vi "PulseOutput.vi"(1 "Pulse Duration (ms)":u32, 2 "Instantaneous Trigger":bool) -> (0 "State Out":bool)   [LabVIEW 2018]
doc: "This VI produces a True pulse of a specified duration when triggered. The external trigger is expected to be instaneous (e.g. from a rising edge trigger). If the trigger is not instantaneous, the pulse will go True immediately but the pulse timmer will not start counting down until the falling edge of the trigger."
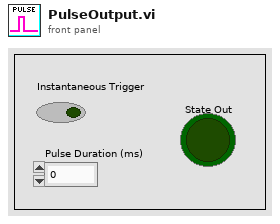
[diagram p1: front panel]
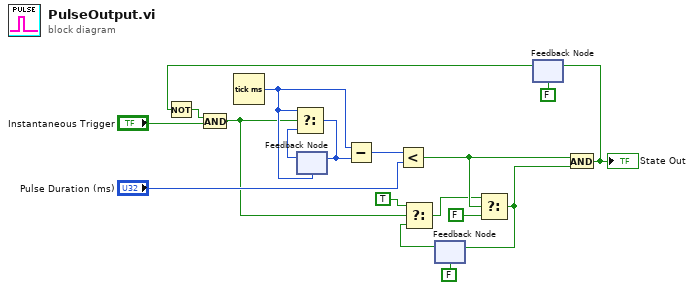
[diagram p0: block diagram]
diagram:
  n1 = Tick Count (ms)() -> (millisecond timer value=w8:u32)
  n2 = feedback #1(w8) -> (w18:u32)
  n3 = feedback #2(FALSE ("f")) -> (w11:bool)
  n4 = feedback #3(FALSE) -> (w2:bool)
  n5 = Not(x=w2) -> (.not. x?=w3:bool)
  n6 = And(x=w3, y="Instantaneous Trigger") -> (x .and. y?=w5:bool)
  n7 = Select(t=w8, s=w5, f=w18) -> (s? t:f=w7:u32)
  n8 = feedback-in #1(w7) -> ()
  n9 = Subtract(x=w8, y=w7) -> (x-y=w17:u32)
  n10 = Less?(x=w17, y="Pulse Duration (ms)") -> (x < y?=w14:bool)
  n11 = Select(t=TRUE, s=w5, f=w11) -> (s? t:f=w13:bool)
  n12 = Select(t=w13, s=w14, f=FALSE) -> (s? t:f=w9:bool)
  n13 = feedback-in #2(w9) -> ()
  n14 = And(x=w14, y=w9) -> (x .and. y?=w4:bool)
  "State Out" <- w4
  n15 = feedback-in #3(w4) -> ()
